vi "_getChannelLength.vi"(4 "error in (no error)":errorcluster, 7 "channel refnum in":refnum<k20>) -> (0 "error out":errorcluster, 2 "channel length":i32, 3 "channel refnum out":refnum<k20>)   [LabVIEW 2017]
uses:
  <vilib>/Platform/storage/Storage.llb/__loadPropRefList.vi
  <vilib>/Platform/storage/Storage.llb/__loadPropInt32.vi
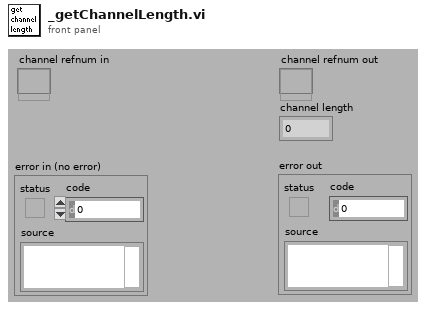
[diagram p1: front panel]
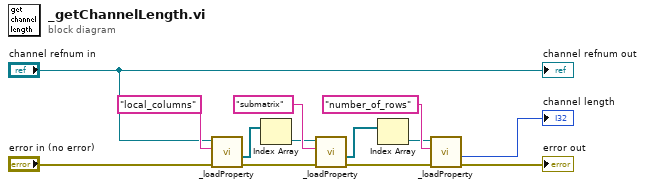
[diagram p0: block diagram]
diagram:
  n1 = call-poly <vilib>:"_loadProperty.vi"("error in (no error)"="error in (no error)", "Property name"="local_columns", "storage refnum"="channel refnum in") -> ("error out"=w10:errorcluster, "Value"=w3:refnum<k20>[])  [unwired: 6 in, 1 out]
  n2 = Index Array(array=w3) -> (element=w4:refnum<k20>)  [unwired: 1 in]
  n3 = call-poly <vilib>:"_loadProperty.vi"("error in (no error)"=w10, "Property name"="submatrix", "storage refnum"=w4) -> ("error out"=w11:errorcluster, "Value"=w6:refnum<k20>[])  [unwired: 6 in, 1 out]
  n4 = Index Array(array=w6) -> (element=w7:refnum<k20>)  [unwired: 1 in]
  n5 = call-poly <vilib>:"_loadProperty.vi"("error in (no error)"=w11, "Property name"="number_of_rows", "storage refnum"=w7) -> ("error out"=→"error out":errorcluster, "Value"=→"channel length":i32)  [unwired: 6 in, 1 out]
  "channel refnum out" <- "channel refnum in"
